vi "entry type constant.vi"() -> (0 "map":T1)   [LabVIEW 2024, in "status manager.lvlib"]
uses:
  status manager.lvlib
  collection type.ctl
  entry type.ctl
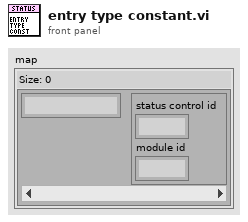
[diagram p1: front panel]
types:
  T1 = typedef "status manager.lvlib/collection type.ctl" = map{string, T2}
  T2 = typedef "status manager.lvlib/entry type.ctl" = cluster{"status control id":i32, "module id":i32}
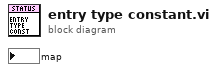
[diagram p0: block diagram]
diagram:
